vi "ABB make pass-Fail criteria.vi"(0 "Loads (% Rated)":dbl[](array[numeric]), 1 "Efficiency Readings":dbl[][](array[numeric]) format="%#_4g", 2 "spect temp rise":cluster{"Stator":string, "Rotor":string}, 3 "motor type":i32, 5 "Load selection":bool[](array[boolean]), 7 "Specified Efficiencies (%)":dbl[](array[numeric])=[0.0, 0.0, 0.0, 0.0], 9 "Partial load":cluster{" Stator dT":dbl, "Rotor dT":dbl}, 11 "Temperature Rise Settings":T1, 12 "Rated Data":T2, 14 "Specified  Power Factor":dbl[](array[numeric])=[0.0, 0.0, 0.0, 0.0]) -> (4 "Entries":string[][](array[string]), 6 "row headers":string[](array[string]), 8 "measurements taken":bool[](array[boolean]), 10 "Pass/Fail Criteria":string[][](table))   [LabVIEW 2017]
uses:
  ABB global.vi
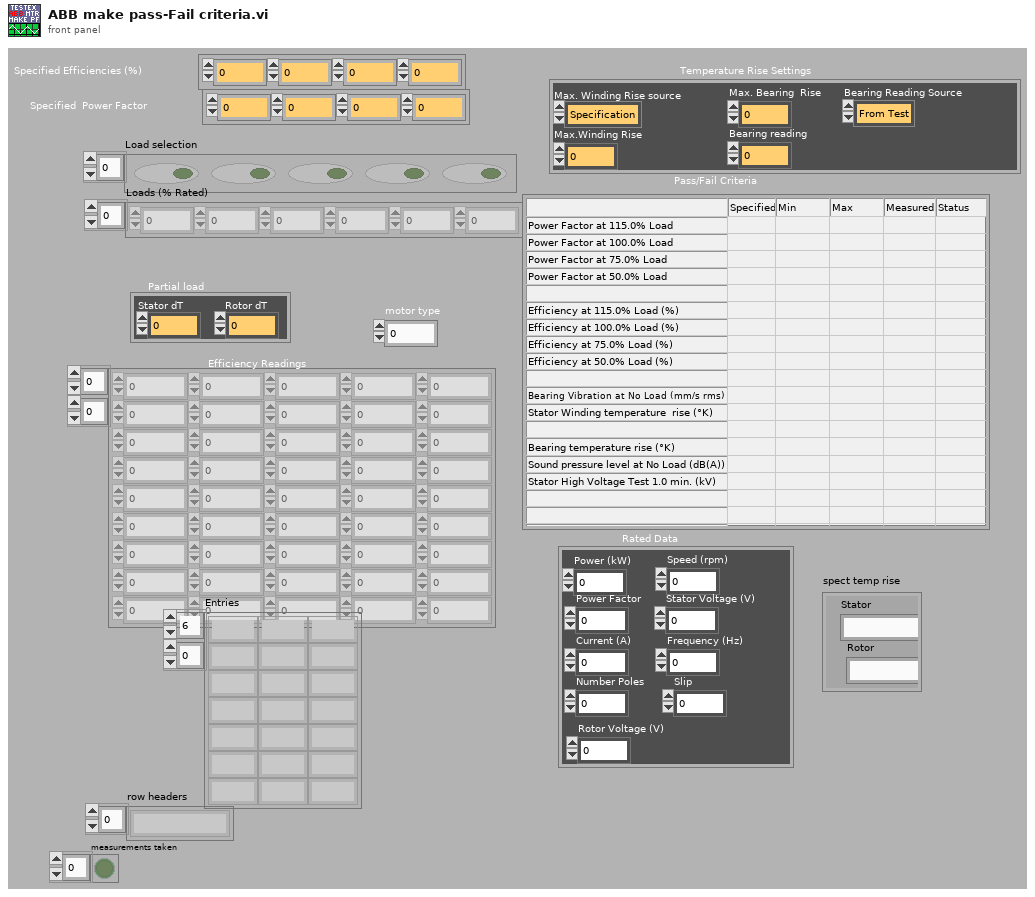
[diagram p1: front panel]
types:
  T1 = cluster{"Max. Winding Rise source":enum16{"Specification", "Enter"}, "Max.Winding Rise":dbl, " Max. Bearing  Rise":dbl, "Bearing Reading Source":enum16{"From Test", "Enter"}, "Bearing reading":dbl}
  T2 = cluster{"Power (kW)":dbl, "Speed (rpm)":dbl, "Power Factor":dbl, "Stator Voltage (V)":dbl, "Current (A)":dbl, "Frequency (Hz)":dbl, "Number Poles":dbl, "Slip":dbl, "Rotor Voltage (V)":dbl}
  T3 = cluster{"Prior to test":dbl, "Prior v":dbl, "Prior temp":dbl, "After test":dbl, "after v":dbl, "After temp":dbl, "Test Voltage (kV)":dbl, "Test Time (min)":dbl}
  T4 = cluster{"Stator R":dbl, "Stator dT":dbl, "Rotor R":dbl, "Rotor dT":dbl, "Stator Cooling curve":dbl[][], "Rotor Cooling curve":dbl[][], "Select Resistance":enum16{"Fitted zero Res.", "Selected Res.", "Entered Res."}}[]
  T5 = cluster{"Stator R":dbl, "Stator dT":dbl, "Rotor R":dbl, "Rotor dT":dbl, "Stator Cooling curve":dbl[][], "Rotor Cooling curve":dbl[][], "Select Resistance":enum16{"Fitted zero Res.", "Selected Res.", "Entered Res."}}
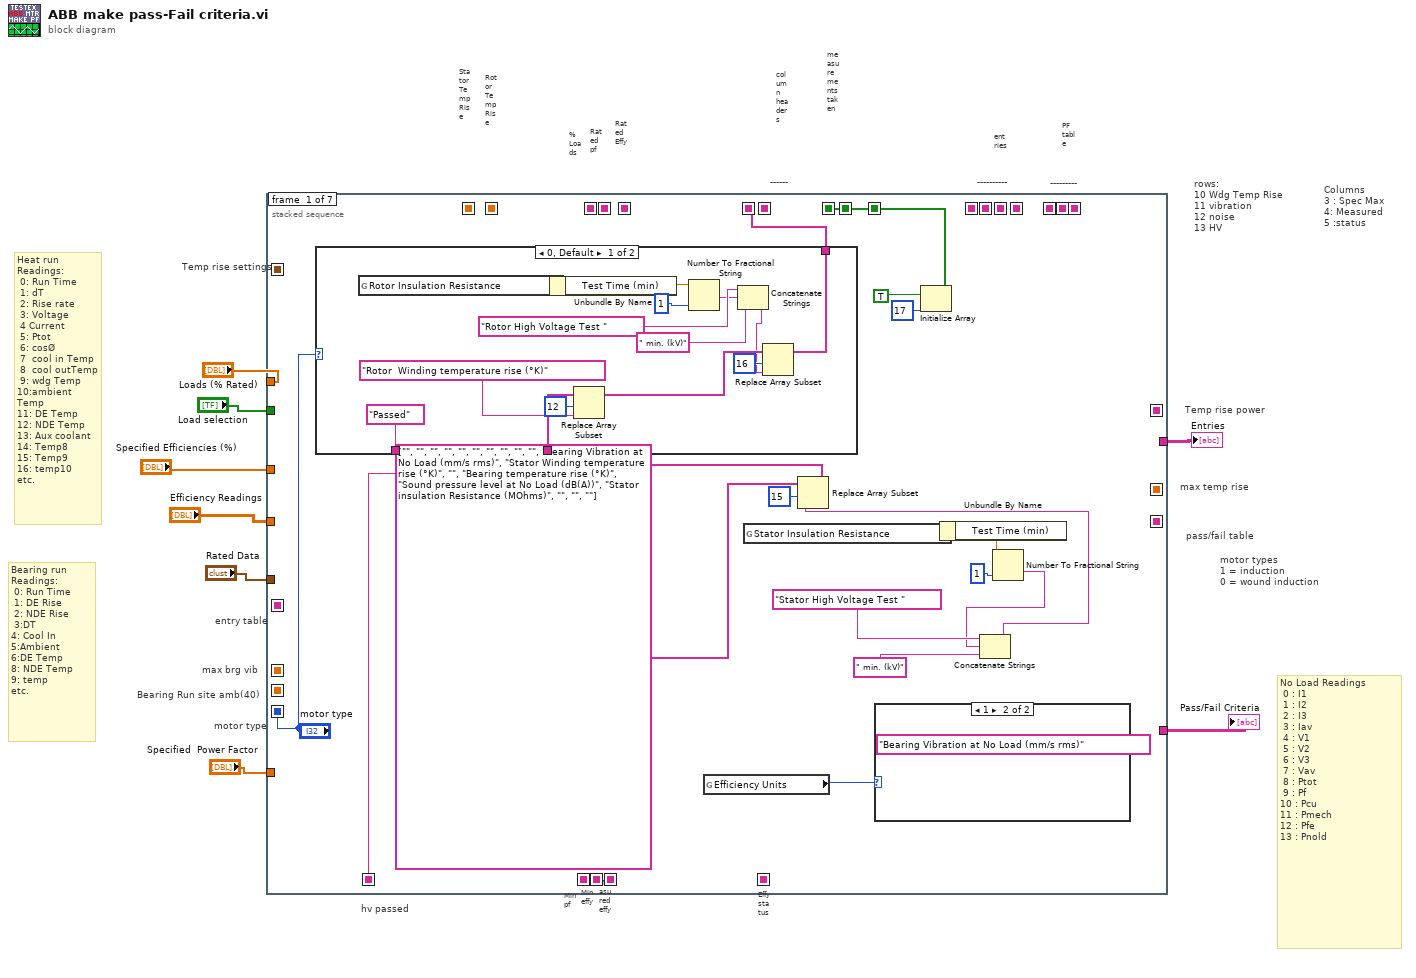
[diagram p0: block diagram]
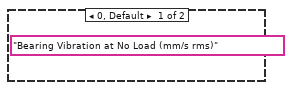
[diagram p2: hidden frame]
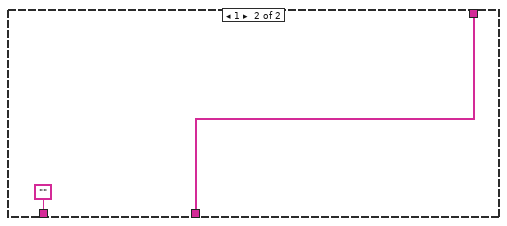
[diagram p3: hidden frame]
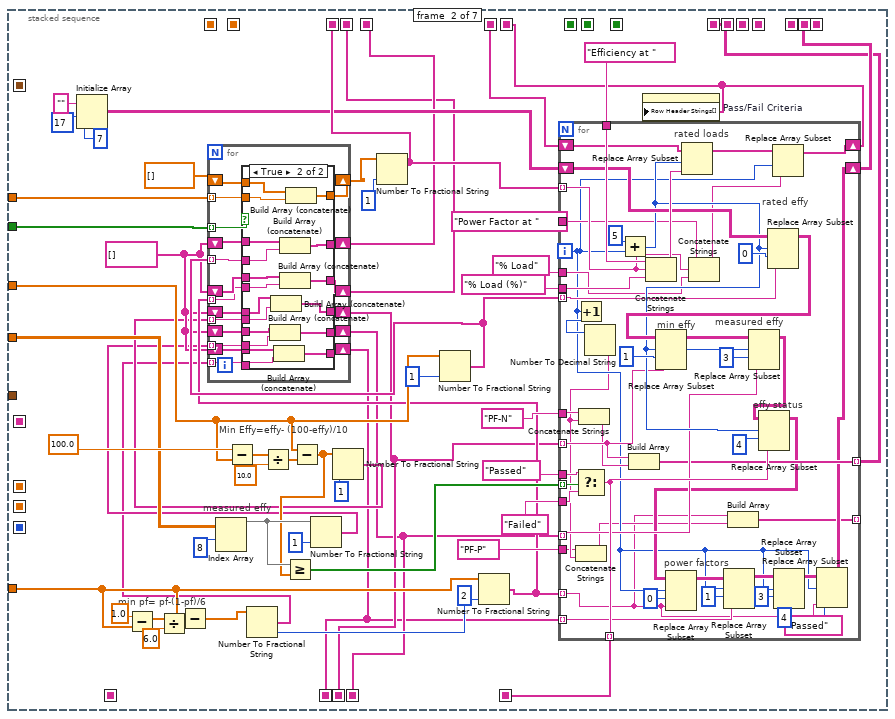
[diagram p4: hidden frame]
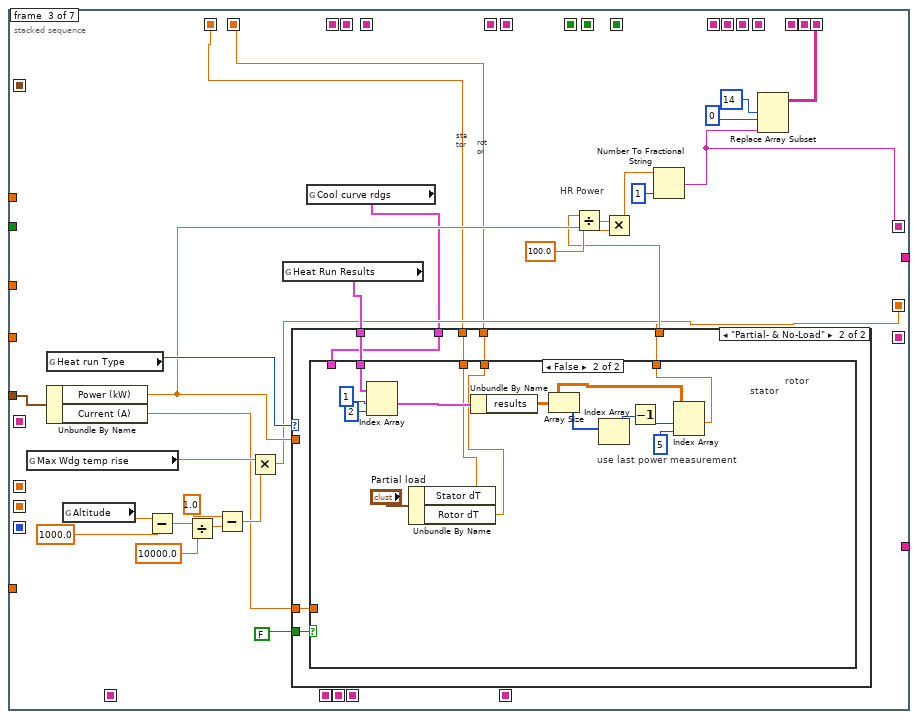
[diagram p6: hidden frame]
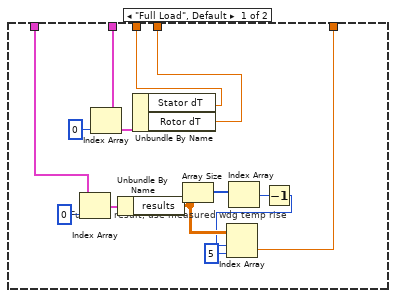
[diagram p7: hidden frame]
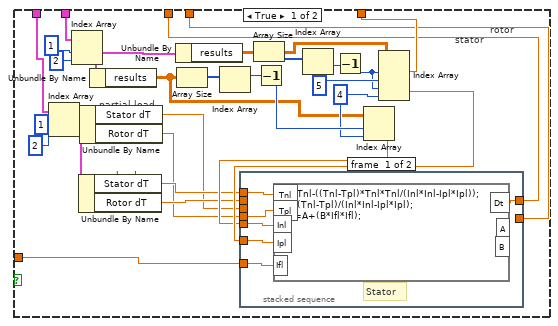
[diagram p8: hidden frame]
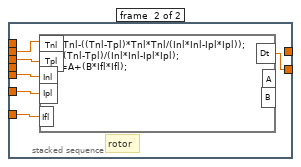
[diagram p9: hidden frame]
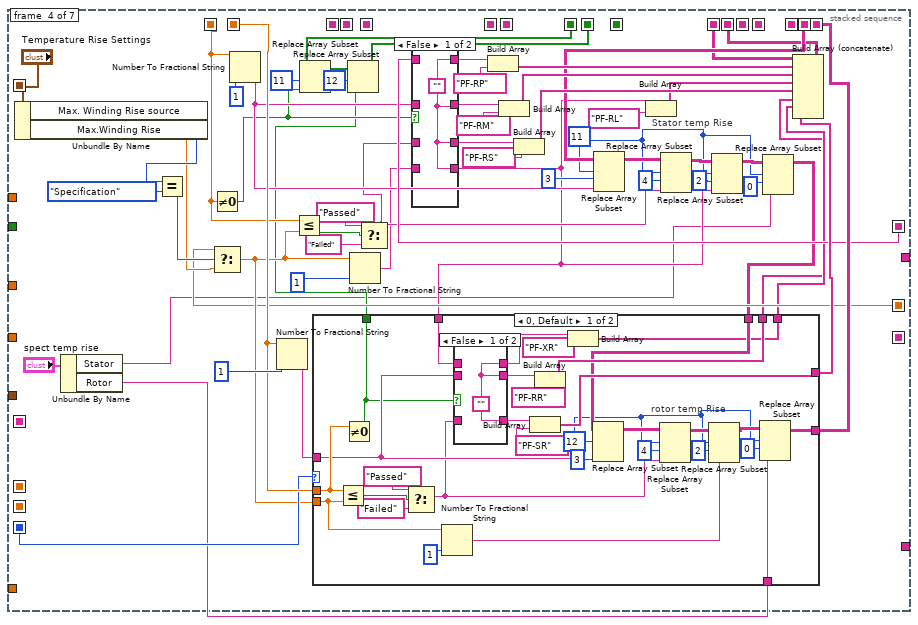
[diagram p10: hidden frame]
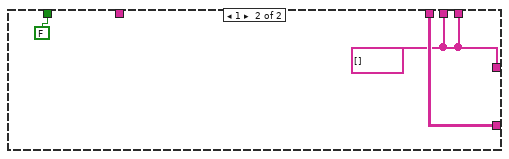
[diagram p13: hidden frame]
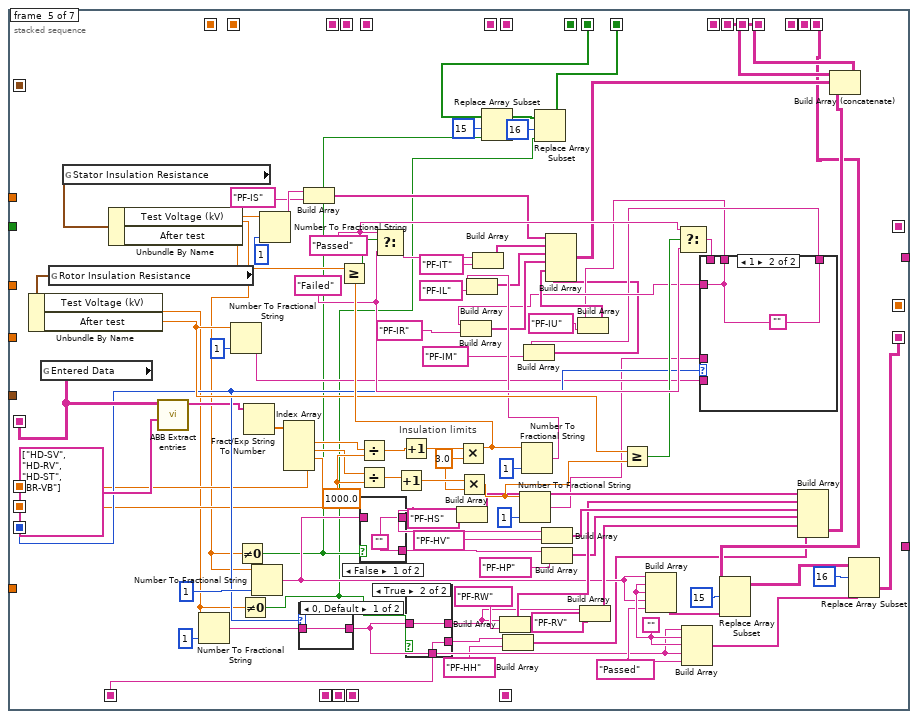
[diagram p14: hidden frame]
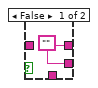
[diagram p15: hidden frame]
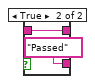
[diagram p16: hidden frame]
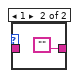
[diagram p17: hidden frame]
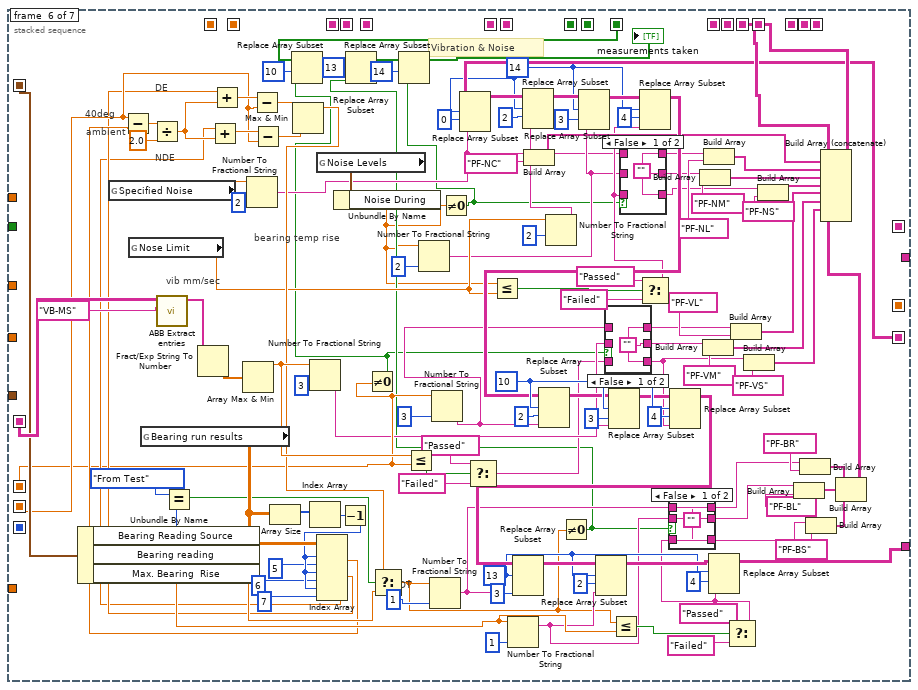
[diagram p19: hidden frame]
diagram:
  # "hv passed"
  # "measurements taken"
  # "Bearing run Readings:\n 0: Run Time\n 1: DE Rise\n 2: NDE Rise\n 3:DT\n4: Cool In\n5:Ambient\n6:DE Temp\n8: NDE Temp\n9: temp\netc."
  # "max brg vib"
  # "Bearing Run site amb(40)"
  # "Temp rise settings"
  # "------"
  # "column headers"
  # "motor type"
  # "PF table"
  # "entries"
  # "---------"
  # "----------"
  # "Rotor Temp Rise"
  # "Stator Temp Rise"
  # "pass/fail table"
  # "entry table"
  # "motor types \n1 = induction\n0 = wound induction"
  # "Temp rise power"
  # "Effy status"
  # "Measured effy"
  # "Min effy"
  # "Min pf"
  # "Rated Effy"
  # "Rated pf"
  # "% Loads"
  # "Columns\n3 : Spec Max\n4: Measured\n5 :status"
  # "rows:\n10 Wdg Temp Rise\n11 vibration\n12 noise\n13 HV"
  # "max temp rise"
  # "No Load Readings\n 0 : I1\n 1 : I2\n 2 : I3\n 3 : Iav\n 4 : V1\n 5 : V2\n 6 : V3\n 7 : Vav\n 8 : Ptot\n 9 : Pf\n10 : Pcu\n11 : Pmech\n12 : Pfe\n13 : Pnold"
  # "Heat run Readings:\n 0: Run Time\n 1: dT\n 2: Rise rate\n 3: Voltage\n 4 Current\n 5: Ptot\n 6: cosØ\n 7  cool in Temp\n 8  cool outTemp\n 9: wdg Temp\n10:ambient Temp\n11: DE Temp\n12: NDE Temp\n13: Aux coolant\n14: Temp8\n15: Temp9\n16: temp10\netc."
  n1 = stacked-sequence {
    seq-local: [_ w83 _ _ _ _ _] -> [_ _ w188 _ _ _ _]
    seq-local: [_ _ w188 _ _ _ _] -> [_ _ _ w330 _ _ _]
    seq-local: [_ _ w193 _ _ _ _] -> [_ _ _ w315 _ _ _]
    seq-local: [_ w73 _ _ _ _ _] -> [_ _ _ _ _ _ w663]
    seq-local: [_ w51 _ _ _ _ _] -> [_ _ _ _ _ _ w635]
    seq-local: [_ w52 _ _ _ _ _] -> [_ _ _ _ _ _ w661]
    seq-local: [_ w42 _ _ _ _ _] -> [_ _ _ _ _ _ w651]
    seq-local: [_ w46 _ _ _ _ _] -> [_ _ _ _ _ _ w657]
    seq-local: [_ w44 _ _ _ _ _] -> [_ _ _ _ _ _ w656]
    seq-local: [_ w72 _ _ _ _ _] -> [_ _ _ _ _ _ w654]
    seq-local: [_ _ _ w324 _ _ _] -> [_ _ _ _ w446 _ _]
    seq-local: [_ _ w192 _ _ _ _] -> [_ _ _ w314 _ _ _]
    seq-local: [_ _ w190 _ _ _ _] -> [_ _ _ w313 _ _ _]
    seq-local: [_ _ _ _ w445 _ _] -> [_ _ _ _ _ w577 _]
    seq-local: [_ _ _ _ w478 _ _] -> [_ _ _ _ _ w586 _]
    seq-local: [_ _ _ _ w450 _ _] -> [_ _ _ _ _ w534 _]
    seq-local: ["motor type" _ _ _ _ _ _] -> [_ _ _ w323 w448 _ _]
    seq-local: [_ _ w189 _ _ _ _] -> [_ _ _ w326 _ _ _]
    seq-local: [_ _ _ w325 _ _ _] -> [_ _ _ _ w415 _ _]
    seq-local: [_ _ _ _ _ w576 _] -> [_ _ _ _ _ _ w644]
    seq-local: [w25 _ _ _ _ _ _] -> [_ w69 _ _ _ _ _]
    seq-local: [_ w68 _ _ _ _ _] -> [_ _ _ _ _ _ w643]
    seq-local: [_ w65 _ _ _ _ _] -> [_ _ _ w322 _ _ _]
    seq-local: [_ _ _ "Temperature Rise Settings" _ _ _] -> [_ _ _ _ _ w558 _]
    seq-local: [_ _ _ _ w414 _ _] -> [_ _ _ _ _ w545 _]
    seq-local: [_ _ _ _ w413 _ _] -> [_ _ _ _ _ w527 _]
    seq-local: [w11 _ _ _ _ _ _] -> [_ _ _ w305 _ _ _]
    seq-local: [_ _ _ w300 _ _ _] -> [_ _ _ _ w399 _ _]
    seq-local: [_ _ _ _ w397 _ _] -> [_ _ _ _ _ w498 _]
    seq-local: [w10 _ _ _ _ _ _] -> [_ _ _ _ w392 _ _]
    tunnel: [_ _ _ _ _ w573 _] -> w3
    tunnel: "Loads (% Rated)" -> [_ w82 _ _ _ _ _]
    tunnel: "Load selection" -> [_ w81 _ _ _ _ _]
    tunnel: "Efficiency Readings" -> [_ w75 _ _ _ _ _]
    tunnel: "Rated Data" -> [_ _ w213 _ _ _ _]
    tunnel: [_ _ _ _ _ _ w645] -> w4
    tunnel: "Specified  Power Factor" -> [_ w58 _ _ _ _ _]
    tunnel: "Specified Efficiencies (%)" -> [_ w53 _ _ _ _ _]
    frame #0 {
      n2 = global read "ABB global.vi" "Efficiency Units"() -> (w9:u16)
      n3 = global read "ABB global.vi" "Stator Insulation Resistance"() -> (w23:T3)
      n4 = case shown="1" w9 {
        frame 0, Default {
          (unwired) "Bearing Vibration at No Load (mm/s rms)"
        }
        frame 1 {
          (unwired) "Bearing Vibration at No Load (mm/s rms)"
        }
      }
      n5 = Initialize Array(TRUE, 17 ("dimension size")) -> (w11:bool[])
      n6 = Unbundle By Name(w23) -> ("Test Time (min)"=w22:dbl)
      n7 = Number To Fractional String(number=w22, precision (6)=i16 1 ("width (-)")) -> (F-format string=w19:string)  [unwired: 2 in]
      n8 = Concatenate Strings("Stator High Voltage Test ", w19, " min. (kV)") -> (w15:string)
      n9 = Replace Array Subset(array=string[] ["", "", "", "", "", "", "", "", "", "", "Bearing Vibration at No Load (mm/s rms)", "Stator Winding temperature  rise (°K)", "", "Bearing temperature rise (°K)", "Sound pressure level at No Load (dB(A))", "Stator insulation Resistance (MOhms)", "", "", ""], new element=w15, index=15) -> (w16:string[])
      n10 = case shown="0, Default" "motor type" {
        tunnel: w16 -> [w39 w41]
        tunnel: [w27 w41] -> w25
        tunnel: ["Passed" ""] -> w10
        frame 0, Default {
          n11 = global read "ABB global.vi" "Rotor Insulation Resistance"() -> (w34:T3)
          n12 = Unbundle By Name(w34) -> ("Test Time (min)"=w32:dbl)
          n13 = Replace Array Subset(array=w39, new element="Rotor  Winding temperature rise (°K)", index=12) -> (w35:string[])
          n14 = Number To Fractional String(number=w32, precision (6)=i16 1 ("width (-)")) -> (F-format string=w30:string)  [unwired: 2 in]
          n15 = Concatenate Strings("Rotor High Voltage Test ", w30, " min. (kV)") -> (w28:string)
          n16 = Replace Array Subset(array=w35, new element=w28, index=16) -> (w27:string[])
        }
        frame 1 {
        }
      }
    }
    frame #1 {
      w48 = string[] []
      w56 = i16 2 ("precision (6)")
      # "min pf= pf-(1-pf)/6"
      # "measured effy"
      # "Min Effy=effy- (100-effy)/10"
      n17 = Initialize Array("" ("element"), 17 ("dimension size"), 7 ("dimension size")) -> (w55:string[][])
      n18 = Subtract(x=1.0, y=w58) -> (x-y=w61:dbl[])
      n19 = Divide(x=w61, y=6.0) -> (x/y=w59:dbl[])
      n20 = Subtract(x=w58, y=w59) -> (x-y=w57:dbl[])
      n21 = Index Array(array=w75, index (row)=8 ("disabled index (col)")) -> (element=w79:dbl[])  [unwired: 1 in]
      n22 = Subtract(x=100.0, y=w53) -> (x-y=w87:dbl[])
      n23 = Number To Fractional String(number=w57, precision (6)=w56) -> (F-format string=w43:string[])  [unwired: 2 in]
      n24 = Divide(x=w87, y=10.0) -> (x/y=w85:dbl[])
      n25 = Subtract(x=w53, y=w85) -> (x-y=w67:dbl[])
      n26 = Greater Or Equal?(x=w79, y=w67) -> (x >= y?=w78:bool[])
      n27 = Number To Fractional String(number=w79, precision (6)=i16 1) -> (F-format string=w45:string[])  [unwired: 2 in]
      n28 = Number To Fractional String(number=w67, precision (6)=i16 1) -> (F-format string=w47:string[])  [unwired: 2 in]
      n29 = Number To Fractional String(number=w53, precision (6)=i16 1) -> (F-format string=w50:string[])  [unwired: 2 in]
      n30 = Number To Fractional String(number=w58, precision (6)=w56) -> (F-format string=w49:string[])  [unwired: 2 in]
      n31 = for {
        tunnel: w81 -> [w162] mode=indexing
        tunnel: w82 -> [w161] mode=indexing
        shift-right: [w160] -> w91
        shift-left: dbl[] [] -> [w159]
        shift-right: [w157] -> w52
        shift-left: w48 -> [w158]
        shift-right: [w155] -> w51
        shift-left: w48 -> [w156]
        tunnel: w50 -> [w154] mode=indexing
        tunnel: w49 -> [w153] mode=indexing
        shift-right: [w146] -> w46
        shift-left: w48 -> [w148]
        shift-right: [w149] -> w44
        shift-left: w48 -> [w150]
        shift-right: [w151] -> w42
        shift-left: w48 -> [w152]
        tunnel: w47 -> [w147] mode=indexing
        tunnel: w45 -> [w145] mode=indexing
        tunnel: w43 -> [w144] mode=indexing
        n32 = case shown="True" w162 {
          tunnel: w161 -> [_ w186]
          tunnel: [w168 w185] -> w160
          tunnel: w159 -> [w168 w184]
          tunnel: w158 -> [w167 w183]
          tunnel: [w167 w182] -> w157
          tunnel: w156 -> [w166 w181]
          tunnel: [w166 w178] -> w155
          tunnel: w154 -> [_ w180]
          tunnel: w153 -> [_ w179]
          tunnel: w152 -> [w163 w177]
          tunnel: [w163 w176] -> w151
          tunnel: w150 -> [w164 w175]
          tunnel: [w164 w174] -> w149
          tunnel: w148 -> [w165 w173]
          tunnel: w147 -> [_ w172]
          tunnel: [w165 w171] -> w146
          tunnel: w145 -> [_ w170]
          tunnel: w144 -> [_ w169]
          frame False {
          }
          frame True {
            n33 = Build Array (concatenate)(w175, w170) -> (w174:string[])
            n34 = Build Array (concatenate)(w173, w172) -> (w171:string[])
            n35 = Build Array (concatenate)(w177, w169) -> (w176:string[])
            n36 = Build Array (concatenate)(w183, w180) -> (w182:string[])
            n37 = Build Array (concatenate)(w181, w179) -> (w178:string[])
            n38 = Build Array (concatenate)(w184, w186) -> (w185:dbl[])
          }
        }
      }
      n39 = Number To Fractional String(number=w91, precision (6)=i16 1) -> (F-format string=w73:string[])  [unwired: 2 in]
      n40 = for {
        tunnel: w73 -> [w115] mode=indexing
        shift-right: [w101] -> w83
        shift-left: w55 -> [w128]
        tunnel: w50 -> [w125] mode=indexing
        tunnel: w46 -> [w121] mode=indexing
        tunnel: w44 -> [w124] mode=indexing
        tunnel: w78 -> [w139] mode=indexing
        tunnel: "Passed" -> [w138]
        tunnel: "Failed" -> [w137]
        tunnel: [w135] -> w72 mode=indexing
        tunnel: "Efficiency at " -> [w131]
        tunnel: "% Load (%)" ("string") -> [w130]
        shift-right: [w117] -> w68
        shift-left: w69 -> [w127]
        tunnel: "PF-N" -> [w122]
        tunnel: [w119] -> w65 mode=indexing
        tunnel: "% Load" ("string") -> [w116]
        tunnel: "Power Factor at " -> [w114]
        tunnel: w49 -> [w97] mode=indexing
        tunnel: w42 -> [w112] mode=indexing
        tunnel: "PF-P" -> [w99]
        tunnel: [w96] -> _ mode=indexing
        i -> [w104]
        # "power factors"
        # "effy status"
        # "measured effy"
        # "min effy"
        # "rated effy"
        # "rated loads"
        n41 = Increment(x=w104) -> (x+1=w123:i32)
        n42 = Select(t=w138, s=w139, f=w137) -> (s? t:f=w135:string)
        n43 = Number To Decimal String(number=w123) -> (decimal integer string=w100:string)  [unwired: 1 in]
        n44 = Concatenate Strings(w99, w100) -> (w98:string)
        n45 = Concatenate Strings(w122, w100) -> (w120:string)
        n46 = Add(x=5 ("disabled index (col)"), y=w104) -> (x+y=w126:i32)
        n47 = Build Array(w121, w120) -> (w119:string[])
        n48 = Concatenate Strings(w131, w115, w130) -> (w132:string)
        n49 = Replace Array Subset(array=w127, new element=w132, index=w126) -> (w118:string[])
        n50 = Concatenate Strings(w114, w115, w116) -> (w113:string)
        n51 = Build Array(w97, w98) -> (w96:string[])
        n52 = Replace Array Subset(array=w128, new element=w125, index (row)=w126, index (col)=0 ("disabled index (col)")) -> (w129:string[][])
        n53 = Replace Array Subset(array=w129, new element=w121, index (row)=w126, index (col)=1 ("disabled index (col)")) -> (w133:string[][])
        n54 = Replace Array Subset(array=w133, new element=w124, index (row)=w126, index (col)=3 ("disabled index (col)")) -> (w134:string[][])
        n55 = Replace Array Subset(array=w134, new element=w135, index (row)=w126, index (col)=4 ("disabled index (col)")) -> (w110:string[][])
        n56 = Replace Array Subset(array=w110, new element=w97, index (row)=w104, index (col)=0 ("disabled index (col)")) -> (w111:string[][])
        n57 = Replace Array Subset(array=w111, new element=w112, index (row)=w104, index (col)=1 ("disabled index (col)")) -> (w108:string[][])
        n58 = Replace Array Subset(array=w118, new element=w113, index=w104) -> (w117:string[])
        n59 = Replace Array Subset(array=w108, new element=w97, index (row)=w104, index (col)=3 ("disabled index (col)")) -> (w105:string[][])
        n60 = Replace Array Subset(array=w105, new element="Passed" ("new element/subarray"), index (row)=w104, index (col)=4 ("disabled index (col)")) -> (w101:string[][])
      }
      n61 = property on="Pass/Fail Criteria" class="Tbl (strict)"("Row Header Strings[]"=w68) -> ()  [unwired: 2 in, 2 out]
    }
    frame #2 {
      # "rotor"
      # "stator"
      # "HR Power"
      n62 = global read "ABB global.vi" "Max Wdg temp rise"() -> (w200:dbl)
      n63 = global read "ABB global.vi" "Heat run Type"() -> (w198:enum16{"Full Load", "Partial- & No-Load"})
      n64 = Unbundle By Name(w213) -> ("Power (kW)"=w196:dbl, "Current (A)"=w194:dbl)
      n65 = global read "ABB global.vi" "Altitude"() -> (w206:dbl)
      n66 = Subtract(x=w206, y=1000.0) -> (x-y=w204:dbl)
      n67 = Divide(x=w204, y=10000.0) -> (x/y=w202:dbl)
      n68 = Subtract(x=1.0, y=w202) -> (x-y=w199:dbl)
      n69 = Multiply(x=w200, y=w199) -> (x*y=w193:dbl)
      n70 = global read "ABB global.vi" "Heat Run Results"() -> (w197:cluster{"results":dbl[][], "Comments":string}[])
      n71 = global read "ABB global.vi" "Cool curve rdgs"() -> (w191:T4)
      n72 = case shown="\"Partial- & No-Load\"" w198 {
        tunnel: w197 -> [w227 w234]
        tunnel: w196 -> [_ _]
        tunnel: [w219 w233] -> w195
        tunnel: w194 -> [_ w232]
        tunnel: [w215 w231] -> w192
        tunnel: w191 -> [w217 w230]
        tunnel: [w214 w229] -> w189
        tunnel: FALSE -> [_ w228]
        frame "Full Load", Default {
          # "Full load result, use measured wdg temp rise"
          n73 = Index Array(array=w227, index=0) -> (element=w225:cluster{"results":dbl[][], "Comments":string})
          n74 = Index Array(array=w217, index=0) -> (element=w218:T5)
          n75 = Unbundle By Name(w225) -> ("results"=w223:dbl[][])
          n76 = Unbundle By Name(w218) -> ("Stator dT"=w215:dbl, "Rotor dT"=w214:dbl)
          n77 = Array Size(array=w223) -> (size(s)=w222:i32[])
          n78 = Index Array(array=w222) -> (element=w220:i32)  [unwired: 1 in]
          n79 = Decrement(x=w220) -> (x-1=w221:i32)
          n80 = Index Array(array=w223, index (row)=w221, index (col)=5 ("disabled index (col)")) -> (element=w219:dbl)
        }
        frame "Partial- & No-Load" {
          n81 = case shown="False" w228 {
            tunnel: w234 -> [w259 w284]
            tunnel: [w258 w283] -> w233
            tunnel: w232 -> [w257 _]
            tunnel: [w256 w278] -> w231
            tunnel: w230 -> [w255 _]
            tunnel: [w235 w277] -> w229
            frame True {
              w242 = 4 ("disabled index (col)")
              # "rotor"
              # "stator"
              # "partial load"
              # "no load"
              n82 = Index Array(array=w255, index #1=1 ("index"), index #2=2 ("index")) -> (element #1=w254:T5, element #2=w251:T5)
              n83 = Index Array(array=w259, index #1=1 ("index"), index #2=2 ("index")) -> (element #1=w263:cluster{"results":dbl[][], "Comments":string}, element #2=w246:cluster{"results":dbl[][], "Comments":string})
              n84 = Unbundle By Name(w251) -> ("Stator dT"=w239:dbl, "Rotor dT"=w238:dbl)
              n85 = Unbundle By Name(w254) -> ("Stator dT"=w237:dbl, "Rotor dT"=w236:dbl)
              n86 = Unbundle By Name(w246) -> ("results"=w240:dbl[][])
              n87 = Unbundle By Name(w263) -> ("results"=w248:dbl[][])
              n88 = Array Size(array=w240) -> (size(s)=w245:i32[])
              n89 = Index Array(array=w245) -> (element=w244:i32)  [unwired: 1 in]
              n90 = Array Size(array=w248) -> (size(s)=w261:i32[])
              n91 = Decrement(x=w244) -> (x-1=w243:i32)
              n92 = Index Array(array=w261) -> (element=w260:i32)  [unwired: 1 in]
              n93 = Decrement(x=w260) -> (x-1=w250:i32)
              n94 = Index Array(array=w240, index (row)=w243, index (col)=w242) -> (element=w241:dbl)
              n95 = Index Array(array=w248, index (row) #1=w250, index (col) #1=5 ("disabled index (col)"), index (row) #2=w250, index (col) #2=w242) -> (element #1=w258:dbl, element #2=w249:dbl)
              n96 = stacked-sequence {
                tunnel: w257 -> [w270 w276]
                tunnel: [w269 _] -> w256
                tunnel: w237 -> [_ w275]
                tunnel: w239 -> [w268 _]
                tunnel: w249 -> [w267 w274]
                tunnel: w241 -> [w266 w273]
                tunnel: [_ w272] -> w235
                tunnel: w238 -> [_ w271]
                tunnel: w236 -> [w265 _]
                frame #0 {
                  # "Stator"
                  n97 = formula code="A=Tnl-((Tnl-Tpl)*Tnl*Tnl/(Inl*Inl-Ipl*Ipl));\nB=(Tnl-Tpl)/(Inl*Inl-Ipl*Ipl);\nDt=A+(B*Ifl*Ifl);"("Tnl"=w268, "Tpl"=w265, "Inl"=w266, "Ipl"=w267, "Ifl"=w270) -> ("Dt"=w269:dbl)  [unwired: 2 out]
                }
                frame #1 {
                  # "rotor"
                  n98 = formula code="A=Tnl-((Tnl-Tpl)*Tnl*Tnl/(Inl*Inl-Ipl*Ipl));\nB=(Tnl-Tpl)/(Inl*Inl-Ipl*Ipl);\nDt=A+(B*Ifl*Ifl);"("Tnl"=w271, "Tpl"=w275, "Inl"=w273, "Ipl"=w274, "Ifl"=w276) -> ("Dt"=w272:dbl)  [unwired: 2 out]
                }
              }
            }
            frame False {
              # "use last power measurement"
              # "rotor"
              # "stator"
              n99 = Index Array(array=w284, index #1=1 ("index"), index #2=2 ("index")) -> (element #1=w288:cluster{"results":dbl[][], "Comments":string})  [unwired: 1 out]
              n100 = Unbundle By Name("Partial load") -> ("Stator dT"=w278:dbl, "Rotor dT"=w277:dbl)
              n101 = Unbundle By Name(w288) -> ("results"=w281:dbl[][])
              n102 = Array Size(array=w281) -> (size(s)=w286:i32[])
              n103 = Index Array(array=w286) -> (element=w285:i32)  [unwired: 1 in]
              n104 = Decrement(x=w285) -> (x-1=w282:i32)
              n105 = Index Array(array=w281, index (row)=w282, index (col)=5 ("disabled index (col)")) -> (element=w283:dbl)
            }
          }
        }
      }
      n106 = Divide(x=w195, y=w196) -> (x/y=w212:dbl)
      n107 = Multiply(x=w212, y=100.0) -> (x*y=w207:dbl)
      n108 = Number To Fractional String(number=w207, precision (6)=i16 1) -> (F-format string=w190:string)  [unwired: 2 in]
      n109 = Replace Array Subset(array=w188, new element=w190, index (row)=14, index (col)=0 ("disabled index (col)")) -> ()  [unwired: 1 out]
    }
    frame #3 {
      w294 = 11 ("index (row)")
      # "Stator temp Rise"
      n110 = Unbundle By Name("Temperature Rise Settings") -> ("Max. Winding Rise source"=w320:enum16{"Specification", "Enter"}, "Max.Winding Rise"=w317:dbl)
      n111 = Unbundle By Name("spect temp rise") -> ("Stator"=w291:string, "Rotor"=w290:string)
      n112 = Equal?(x=w320, y=enum16{"Specification", "Enter"}."Specification") -> (x = y?=w318:bool)
      n113 = Not Equal To 0?(x=w314) -> (x != 0?=w303:bool)
      n114 = Select(t=w315, s=w318, f=w317) -> (s? t:f=w316:dbl)
      n115 = Number To Fractional String(number=w314, precision (6)=i16 1) -> (F-format string=w312:string)  [unwired: 2 in]
      n116 = Number To Fractional String(number=w326, precision (6)=i16 1) -> (F-format string=w329:string)  [unwired: 2 in]
      n117 = Less Or Equal?(x=w314, y=w316) -> (x <= y?=w347:bool)
      n118 = Replace Array Subset(array=w305, new element=w303, index=11) -> (w304:bool[])
      n119 = Number To Fractional String(number=w316, precision (6)=i16 1) -> (F-format string=w310:string)  [unwired: 2 in]
      n120 = Select(t="Passed", s=w347, f="Failed") -> (s? t:f=w311:string)
      n121 = case shown="False" w303 {
        tunnel: w313 -> [_ w353]
        tunnel: w312 -> [_ w352]
        tunnel: w311 -> [_ w351]
        tunnel: w310 -> [_ w350]
        tunnel: [w349 w353] -> w309
        tunnel: [w349 w352] -> w308
        tunnel: [w349 w351] -> w307
        tunnel: [w349 w350] -> w306
        frame False {
          w349 = ""
        }
        frame True {
        }
      }
      n122 = Build Array(w309, "PF-RP") -> (w335:string[])
      n123 = Build Array(w308, "PF-RM") -> (w340:string[])
      n124 = Build Array(w307, "PF-RS" ("element")) -> (w339:string[])
      n125 = Replace Array Subset(array=w330, new element=w312, index (row)=w294, index (col)=3 ("disabled index (col)")) -> (w344:string[][])
      n126 = Build Array(w306, "PF-RL" ("element")) -> (w338:string[])
      n127 = Replace Array Subset(array=w344, new element=w311, index (row)=w294, index (col)=4 ("disabled index (col)")) -> (w334:string[][])
      n128 = Replace Array Subset(array=w334, new element=w306, index (row)=w294, index (col)=2 ("disabled index (col)")) -> (w296:string[][])
      n129 = Replace Array Subset(array=w296, new element=w291, index (row)=w294, index (col)=0 ("disabled index (col)")) -> (w295:string[][])
      n130 = case shown="0, Default" w323 {
        tunnel: w329 -> [w364 _]
        tunnel: [w372 w390] -> w297
        tunnel: [w371 w390] -> w327
        tunnel: w295 -> [w370 w391]
        tunnel: w316 -> [w369 _]
        tunnel: w326 -> [w366 _]
        tunnel: [w357 w391] -> w325
        tunnel: [w367 w390] -> w298
        tunnel: w306 -> [w365 _]
        tunnel: [w359 FALSE] -> w299
        tunnel: w290 -> [w354 _]
        frame 0, Default {
          w356 = 12 ("index (row)")
          # "rotor temp Rise"
          n131 = Less Or Equal?(x=w366, y=w369) -> (x <= y?=w374:bool)
          n132 = Not Equal To 0?(x=w366) -> (x != 0?=w359:bool)
          n133 = Select(t="Passed", s=w374, f="Failed") -> (s? t:f=w363:string)
          n134 = Number To Fractional String(number=w369, precision (6)=i16 1) -> (F-format string=w384:string)  [unwired: 2 in]
          n135 = case shown="False" w359 {
            tunnel: w365 -> [_ w388]
            tunnel: [w385 w388] -> w362
            tunnel: w364 -> [_ w387]
            tunnel: w363 -> [_ w386]
            tunnel: [w385 w387] -> w361
            tunnel: [w385 w386] -> w360
            frame False {
              w385 = ""
            }
            frame True {
            }
          }
          n136 = Build Array(w360, "PF-SR" ("element")) -> (w371:string[])
          n137 = Build Array(w361, "PF-RR") -> (w372:string[])
          n138 = Build Array(w362, "PF-XR") -> (w367:string[])
          n139 = Replace Array Subset(array=w370, new element=w364, index (row)=w356, index (col)=3 ("disabled index (col)")) -> (w377:string[][])
          n140 = Replace Array Subset(array=w377, new element=w363, index (row)=w356, index (col)=4 ("disabled index (col)")) -> (w381:string[][])
          n141 = Replace Array Subset(array=w381, new element=w384, index (row)=w356, index (col)=2 ("disabled index (col)")) -> (w358:string[][])
          n142 = Replace Array Subset(array=w358, new element=w354, index (row)=w356, index (col)=0 ("disabled index (col)")) -> (w357:string[][])
        }
        frame 1 {
          w390 = string[] []
        }
      }
      n143 = Replace Array Subset(array=w304, new element=w299, index=12) -> (w300:bool[])
      n144 = Build Array (concatenate)(w322, w335, w340, w338, w339, w297, w298, w327) -> (w324:string[][])
    }
    frame #4 {
      w421 = "Passed" ("element")
      w441 = ""
      w462 = "Failed"
      w469 = 3.0 ("y")
      w474 = 1000.0 ("y")
      w463 = "Passed" ("new element/subarray")
      # "Insulation limits"
      n145 = global read "ABB global.vi" "Entered Data"() -> (w478:string[][])
      n146 = global read "ABB global.vi" "Rotor Insulation Resistance"() -> (w480:T3)
      n147 = Unbundle By Name(w480) -> ("Test Voltage (kV)"=w406:dbl, "After test"=w457:dbl)
      n148 = global read "ABB global.vi" "Stator Insulation Resistance"() -> (w485:T3)
      n149 = Unbundle By Name(w485) -> ("Test Voltage (kV)"=w412:dbl, "After test"=w458:dbl)
      n150 = call "ABB Extract entries.vi"("Entry IDs"=string[] ["HD-SV", "HD-RV", "HD-ST", "BR-VB"], "Entry table in"=w478) -> ("Selected Entries"=w423:string[])  [unwired: 9 in]
      n151 = Number To Fractional String(number=w406, precision (6)=i16 1) -> (F-format string=w447:string)  [unwired: 2 in]
      n152 = Number To Fractional String(number=w457, precision (6)=i16 1) -> (F-format string=w434:string)  [unwired: 2 in]
      n153 = Not Equal To 0?(x=w412) -> (x != 0?=w396:bool)
      n154 = Not Equal To 0?(x=w406) -> (x != 0?=w395:bool)
      n155 = Fract/Exp String To Number(string=w423) -> (number=w476:dbl[])  [unwired: 3 in, 1 out]
      n156 = Number To Fractional String(number=w412, precision (6)=i16 1) -> (F-format string=w410:string)  [unwired: 2 in]
      n157 = Number To Fractional String(number=w458, precision (6)=i16 1) -> (F-format string=w483:string)  [unwired: 2 in]
      n158 = Index Array(array=w476) -> (element #1=w475:dbl, element #2=w459:dbl, element #3=w414:dbl, element #4=w413:dbl)  [unwired: 4 in]
      n159 = case shown="0, Default" w448 {
        tunnel: w447 -> [w492 _]
        tunnel: [w492 ""] -> w405
        frame 0, Default {
        }
        frame 1 {
        }
      }
      n160 = Build Array(w483, "PF-IS") -> (w440:string[])
      n161 = Divide(x=w475, y=w474) -> (x/y=w473:dbl)
      n162 = Divide(x=w459, y=w474) -> (x/y=w472:dbl)
      n163 = case shown="False" w396 {
        tunnel: w410 -> [_ w491]
        tunnel: [w489 w491] -> w409
        tunnel: [w489 "Passed"] -> w408
        frame False {
          w489 = ""
        }
        frame True {
        }
      }
      n164 = Increment(x=w472) -> (x+1=w470:dbl)
      n165 = Increment(x=w473) -> (x+1=w471:dbl)
      n166 = case shown="True" w395 {
        tunnel: w405 -> [_ w488]
        tunnel: [w486 w488] -> w404
        tunnel: [w486 w487] -> w402
        tunnel: w392 -> [_ w487]
        frame False {
          w486 = ""
        }
        frame True {
        }
      }
      n167 = Build Array(w409, "PF-HS" ("element")) -> (w417:string[])
      n168 = Multiply(x=w471, y=w469) -> (x*y=w466:dbl)
      n169 = Greater Or Equal?(x=w458, y=w466) -> (x >= y?=w465:bool)
      n170 = Select(t=w463, s=w465, f=w462) -> (s? t:f=w464:string)
      n171 = Multiply(x=w470, y=w469) -> (x*y=w461:dbl)
      n172 = Build Array(w464, "PF-IT") -> (w439:string[])
      n173 = Replace Array Subset(array=w399, new element=w396, index=15) -> (w398:bool[])
      n174 = Build Array(w404, "PF-RW" ("element")) -> (w416:string[])
      n175 = Build Array(w402, "PF-HH" ("element")) -> (w400:string[])
      n176 = Number To Fractional String(number=w461, precision (6)=i16 1) -> (F-format string=w401:string)  [unwired: 2 in]
      n177 = Number To Fractional String(number=w466, precision (6)=i16 1) -> (F-format string=w438:string)  [unwired: 2 in]
      n178 = Build Array(w438, "PF-IL" ("element")) -> (w436:string[])
      n179 = Replace Array Subset(array=w398, new element=w395, index=16) -> (w397:bool[])
      n180 = Build Array(w409, "PF-HV" ("element")) -> (w426:string[])
      n181 = Build Array(w408, "PF-HP" ("element")) -> (w407:string[])
      n182 = Build Array(w404, "PF-RV" ("element")) -> (w425:string[])
      n183 = Greater Or Equal?(x=w457, y=w461) -> (x >= y?=w460:bool)
      n184 = Build Array(w410, w441, w441, w410, w421) -> (w454:string[])
      n185 = Select(t=w463, s=w460, f=w462) -> (s? t:f=w442:string)
      n186 = Build Array(w405, w441, w441, w405, w421) -> (w449:string[])
      n187 = case shown="1" w448 {
        tunnel: w401 -> [w496 _]
        tunnel: [w496 w497] -> w430
        tunnel: w442 -> [w495 _]
        tunnel: [w495 w497] -> w428
        tunnel: w434 -> [w494 _]
        tunnel: [w494 w497] -> w431
        frame 0, Default {
        }
        frame 1 {
          w497 = ""
        }
      }
      n188 = Build Array(w431, "PF-IR") -> (w433:string[])
      n189 = Build Array(w430, "PF-IM" ("element")) -> (w422:string[])
      n190 = Build Array(w428, "PF-IU") -> (w432:string[])
      n191 = Build Array(w440, w439, w436, w433, w432, w422) -> (w435:string[][])
      n192 = Replace Array Subset(array=w415, new element=w454, index (row)=15) -> (w452:string[][])  [unwired: 1 in]
      n193 = Build Array(w417, w416, w426, w407, w425, w400) -> (w424:string[][])
      n194 = Build Array (concatenate)(w446, w435, w424) -> (w445:string[][])
      n195 = Replace Array Subset(array=w452, new element=w449, index (row)=16) -> (w450:string[][])  [unwired: 1 in]
    }
    frame #5 {
      w571 = 13 ("index (row)")
      w608 = 10 ("index (row)")
      w533 = 14 ("index (row)")
      # "bearing temp rise"
      # "NDE"
      # "DE"
      # "40deg"
      # "ambient"
      # "DT"
      # "Vibration & Noise"
      # "vib mm/sec"
      n196 = Unbundle By Name(w558) -> ("Bearing Reading Source"=w557:enum16{"From Test", "Enter"}, "Bearing reading"=w553:dbl, "Max. Bearing  Rise"=w554:dbl)
      n197 = global read "ABB global.vi" "Specified Noise"() -> (w530:dbl)
      n198 = global read "ABB global.vi" "Nose Limit"() -> (w536:dbl)
      n199 = global read "ABB global.vi" "Bearing run results"() -> (w581:dbl[][])
      n200 = call "ABB Extract entries.vi"("Entry ID"="VB-MS", "Entry table in"=w586) -> ("Selected Entries"=w587:string[])  [unwired: 9 in]
      n201 = Equal?(x=enum16{"From Test", "Enter"}."From Test", y=w557) -> (x = y?=w555:bool)
      n202 = Fract/Exp String To Number(string=w587) -> (number=w613:dbl[])  [unwired: 3 in, 1 out]
      n203 = Array Max & Min(array=w613) -> (max value=w604:dbl)  [unwired: 3 out]
      n204 = Number To Fractional String(number=w530, precision (6)=i16 2) -> (F-format string=w528:string)  [unwired: 2 in]
      n205 = Array Size(array=w581) -> (size(s)=w583:i32[])
      n206 = Number To Fractional String(number=w604, precision (6)=i16 3) -> (F-format string=w525:string)  [unwired: 2 in]
      n207 = Index Array(array=w583) -> (element=w582:i32)  [unwired: 1 in]
      n208 = global read "ABB global.vi" "Noise Levels"() -> (w594:cluster{"Noise Before":dbl, "Noise During":dbl})
      n209 = Unbundle By Name(w594) -> ("Noise During"=w504:dbl)
      n210 = Decrement(x=w582) -> (x-1=w543:i32)
      n211 = Index Array(array=w581, index (row) #1=w543, index (col) #1=5, index (row) #2=w543, index (col) #2=6 ("disabled index (col)"), index (row) #3=w543, index (col) #3=7 ("disabled index (col)")) -> (element #1=w544:dbl, element #2=w541:dbl, element #3=w538:dbl)
      n212 = Subtract(x=w545, y=w544) -> (x-y=w552:dbl)
      n213 = Divide(x=w552, y=2.0) -> (x/y=w550:dbl)
      n214 = Add(x=w538, y=w550) -> (x+y=w548:dbl)
      n215 = Add(x=w541, y=w550) -> (x+y=w549:dbl)
      n216 = Subtract(x=w549, y=w545) -> (x-y=w547:dbl)
      n217 = Subtract(x=w548, y=w545) -> (x-y=w546:dbl)
      n218 = Max & Min(x=w547, y=w546) -> (max(x,y)=w537:dbl)  [unwired: 1 out]
      n219 = Not Equal To 0?(x=w527) -> (x != 0?=w503:bool)
      n220 = Replace Array Subset(array=w498, new element=w503, index=10) -> (w514:bool[])
      n221 = Select(t=w537, s=w555, f=w553) -> (s? t:f=w515:dbl)
      n222 = Less Or Equal?(x=w604, y=w527) -> (x <= y?=w602:bool)
      n223 = Number To Fractional String(number=w504, precision (6)=i16 2) -> (F-format string=w508:string)  [unwired: 2 in]
      n224 = Number To Fractional String(number=w515, precision (6)=i16 1) -> (F-format string=w518:string)  [unwired: 2 in]
      n225 = Number To Fractional String(number=w527, precision (6)=i16 3) -> (F-format string=w526:string)  [unwired: 2 in]
      n226 = Not Equal To 0?(x=w504) -> (x != 0?=w500:bool)
      n227 = Replace Array Subset(array=w534, new element=w528, index (row)=w533, index (col)=0 ("disabled index (col)")) -> (w535:string[][])
      n228 = Select(t="Passed", s=w602, f="Failed") -> (s? t:f=w524:string)
      n229 = Less Or Equal?(x=w504, y=w536) -> (x <= y?=w616:bool)
      n230 = Number To Fractional String(number=w554, precision (6)=i16 1) -> (F-format string=w517:string)  [unwired: 2 in]
      n231 = Build Array(w528, "PF-NC") -> (w511:string[])
      n232 = Number To Fractional String(number=w536, precision (6)=i16 2) -> (F-format string=w507:string)  [unwired: 2 in]
      n233 = Replace Array Subset(array=w535, new element=w507, index (row)=w533, index (col)=2 ("disabled index (col)")) -> (w620:string[][])
      n234 = Not Equal To 0?(x=w515) -> (x != 0?=w513:bool)
      n235 = Replace Array Subset(array=w514, new element=w513, index=13) -> (w502:bool[])
      n236 = Replace Array Subset(array=w502, new element=w500, index=14) -> (→"measurements taken":bool[])
      n237 = Replace Array Subset(array=w620, new element=w508, index (row)=w533, index (col)=3 ("disabled index (col)")) -> (w622:string[][])
      n238 = case shown="False" w503 {
        tunnel: w526 -> [_ w633]
        tunnel: w525 -> [_ w634]
        tunnel: [w631 w634] -> w522
        tunnel: [w631 w633] -> w521
        tunnel: w524 -> [_ w632]
        tunnel: [w631 w632] -> w523
        frame False {
          w631 = ""
        }
        frame True {
          (unwired) "Failed" ("f")
        }
      }
      n239 = Less Or Equal?(x=w515, y=w554) -> (x <= y?=w569:bool)
      n240 = Select(t="Passed", s=w616, f="Failed") -> (s? t:f=w510:string)
      n241 = case shown="False" w500 {
        tunnel: w510 -> [_ w626]
        tunnel: [w623 w626] -> w509
        tunnel: w508 -> [_ w625]
        tunnel: [w623 w625] -> w505
        tunnel: w507 -> [_ w624]
        tunnel: [w623 w624] -> w506
        frame False {
          w623 = ""
        }
        frame True {
        }
      }
      n242 = Replace Array Subset(array=w622, new element=w510, index (row)=w533, index (col)=4 ("disabled index (col)")) -> (w605:string[][])
      n243 = Replace Array Subset(array=w605, new element=w526, index (row)=w608, index (col)=2 ("disabled index (col)")) -> (w607:string[][])
      n244 = Replace Array Subset(array=w607, new element=w525, index (row)=w608, index (col)=3 ("disabled index (col)")) -> (w606:string[][])
      n245 = Replace Array Subset(array=w606, new element=w523, index (row)=w608, index (col)=4 ("disabled index (col)")) -> (w578:string[][])
      n246 = Replace Array Subset(array=w578, new element=w518, index (row)=w571, index (col)=3 ("disabled index (col)")) -> (w575:string[][])
      n247 = Replace Array Subset(array=w575, new element=w517, index (row)=w571, index (col)=2 ("disabled index (col)")) -> (w574:string[][])
      n248 = Build Array(w505, "PF-NM" ("element")) -> (w592:string[])
      n249 = Build Array(w522, "PF-VM" ("element")) -> (w589:string[])
      n250 = Build Array(w506, "PF-NL") -> (w593:string[])
      n251 = Select(t="Passed", s=w569, f="Failed") -> (s? t:f=w516:string)
      n252 = case shown="False" w513 {
        tunnel: w518 -> [_ w630]
        tunnel: w517 -> [_ w629]
        tunnel: w516 -> [_ w628]
        tunnel: [w627 w630] -> _
        tunnel: [w627 w629] -> _
        tunnel: [w627 w628] -> _
        frame False {
          w627 = ""
        }
        frame True {
        }
      }
      n253 = Replace Array Subset(array=w574, new element=w516, index (row)=w571, index (col)=4 ("disabled index (col)")) -> (w573:string[][])
      n254 = Build Array(w521, "PF-VL" ("element")) -> (w590:string[])
      n255 = Build Array(w523, "PF-VS" ("element")) -> (w588:string[])
      n256 = Build Array(w509, "PF-NS" ("element")) -> (w591:string[])
      n257 = Build Array(w517, "PF-BL" ("element")) -> (w561:string[])
      n258 = Build Array(w518, "PF-BR") -> (w562:string[])
      n259 = Build Array(w516, "PF-BS" ("element")) -> (w560:string[])
      n260 = Build Array(w562, w561, w560) -> (w559:string[][])
      n261 = Build Array (concatenate)(w577, w511, w593, w592, w591, w590, w589, w588, w559) -> (w576:string[][])
    }
    frame #6 {
      n262 = for {
        tunnel: "PF-O" -> [w712]
        tunnel: w651 -> [_] mode=indexing
        tunnel: w651 -> [w708] mode=indexing
        tunnel: [w707] -> w650 mode=indexing
        i -> [w713]
        n263 = Increment(x=w713) -> (x+1=w711:i32)
        n264 = Number To Decimal String(number=w711) -> (decimal integer string=w710:string)  [unwired: 1 in]
        n265 = Concatenate Strings(w712, w710) -> (w709:string)
        n266 = Build Array(w708, w709) -> (w707:string[])
      }
      n267 = for {
        tunnel: "PF-L" -> [w726]
        tunnel: w663 -> [w723] mode=indexing
        tunnel: [w721] -> w653 mode=indexing
        i -> [w727]
        n268 = Increment(x=w727) -> (x+1=w725:i32)
        n269 = Number To Decimal String(number=w725) -> (decimal integer string=w724:string)  [unwired: 1 in]
        n270 = Concatenate Strings(w726, w724) -> (w722:string)
        n271 = Build Array(w723, w722) -> (w721:string[])
      }
      n272 = for {
        tunnel: "PF-I" -> [w705]
        tunnel: w657 -> [w701] mode=indexing
        tunnel: [w700] -> w648 mode=indexing
        i -> [w706]
        n273 = Increment(x=w706) -> (x+1=w704:i32)
        n274 = Number To Decimal String(number=w704) -> (decimal integer string=w703:string)  [unwired: 1 in]
        n275 = Concatenate Strings(w705, w703) -> (w702:string)
        n276 = Build Array(w701, w702) -> (w700:string[])
      }
      n277 = for {
        tunnel: "PF-P" -> [w684]
        tunnel: w635 -> [w680] mode=indexing
        tunnel: [w679] -> w641 mode=indexing
        i -> [w685]
        n278 = Increment(x=w685) -> (x+1=w683:i32)
        n279 = Number To Decimal String(number=w683) -> (decimal integer string=w682:string)  [unwired: 1 in]
        n280 = Concatenate Strings(w684, w682) -> (w681:string)
        n281 = Build Array(w680, w681) -> (w679:string[])
      }
      n282 = for {
        tunnel: "PF-F" -> [w677]
        tunnel: w635 -> [w673] mode=indexing
        tunnel: [w672] -> w639 mode=indexing
        i -> [w678]
        n283 = Increment(x=w678) -> (x+1=w676:i32)
        n284 = Number To Decimal String(number=w676) -> (decimal integer string=w675:string)  [unwired: 1 in]
        n285 = Concatenate Strings(w677, w675) -> (w674:string)
        n286 = Build Array(w673, w674) -> (w672:string[])
      }
      n287 = for {
        tunnel: "PF-M" -> [w698]
        tunnel: w656 -> [w695] mode=indexing
        tunnel: [w693] -> w649 mode=indexing
        i -> [w699]
        n288 = Increment(x=w699) -> (x+1=w697:i32)
        n289 = Number To Decimal String(number=w697) -> (decimal integer string=w696:string)  [unwired: 1 in]
        n290 = Concatenate Strings(w698, w696) -> (w694:string)
        n291 = Build Array(w695, w694) -> (w693:string[])
      }
      n292 = for {
        tunnel: "PF-S" -> [w670]
        tunnel: "Passed" ("new element/subarray") -> [w666]
        tunnel: [w665] -> w636 mode=indexing
        tunnel: w635 -> [_] mode=indexing
        i -> [w671]
        n293 = Increment(x=w671) -> (x+1=w669:i32)
        n294 = Number To Decimal String(number=w669) -> (decimal integer string=w668:string)  [unwired: 1 in]
        n295 = Concatenate Strings(w670, w668) -> (w667:string)
        n296 = Build Array(w666, w667) -> (w665:string[])
      }
      n297 = for {
        tunnel: "PF-E" -> [w719]
        tunnel: w661 -> [w715] mode=indexing
        tunnel: [w714] -> w652 mode=indexing
        i -> [w720]
        n298 = Increment(x=w720) -> (x+1=w718:i32)
        n299 = Number To Decimal String(number=w718) -> (decimal integer string=w717:string)  [unwired: 1 in]
        n300 = Concatenate Strings(w719, w717) -> (w716:string)
        n301 = Build Array(w715, w716) -> (w714:string[])
      }
      n302 = for {
        tunnel: "PF-Q" -> [w691]
        tunnel: w654 -> [w688] mode=indexing
        tunnel: [w686] -> w647 mode=indexing
        i -> [w692]
        n303 = Increment(x=w692) -> (x+1=w690:i32)
        n304 = Number To Decimal String(number=w690) -> (decimal integer string=w689:string)  [unwired: 1 in]
        n305 = Concatenate Strings(w691, w689) -> (w687:string)
        n306 = Build Array(w688, w687) -> (w686:string[])
      }
      n307 = Build Array (concatenate)(w653, w641, w639, w652, w650, w649, w648, w636, w647) -> (w646:string[][])
      n308 = Build Array (concatenate)(w644, w646) -> (w645:string[][])
      "row headers" <- w643
    }
  }
  "Pass/Fail Criteria" <- w3
  "Entries" <- w4
